vi "SubVI - Global.vi"() -> ()   [LabVIEW 2017]
panel:
  in  "Datalog Interval":dbl
  in  "Test Info":string[](array[string])
  in  "File Path":path
  in  "Drive Communication Error":bool
  in  "Start Acquisition ?":bool
  in  "Test Aborted":bool
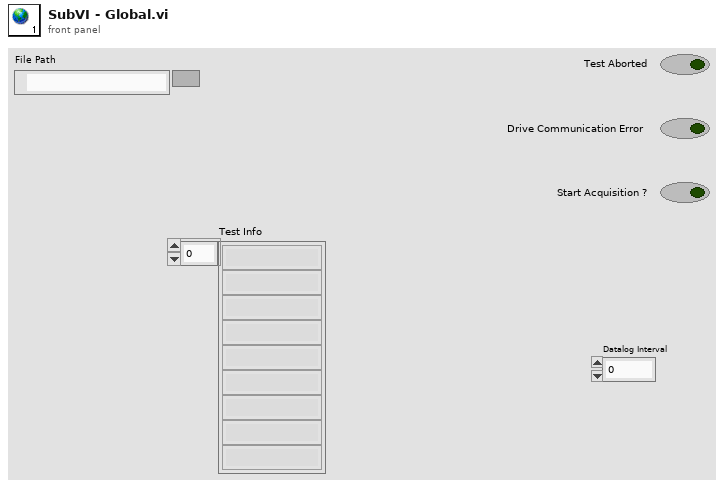
[diagram p1: front panel]
diagram:
